vi "CRYProbe Window Change.vi"(6 "Update Index":i32[](array[numeric]), 8 "Type":enum16{"Curves", "Values", "Results", "WFM"}(ring), 9 "Close Names":string[](array[string]), 10 "Update Names":string[](array[string]), 11 "Probe Type":string) -> ()   [LabVIEW 2013]
uses:
  Global/CRYCurve Library Global.vi
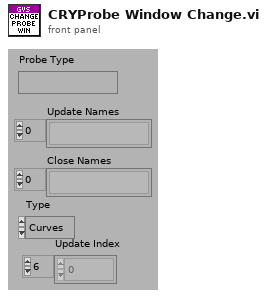
[diagram p1: front panel]
types:
  T1 = cluster{"Type Name":string, "Data Name":string, "Probe VIRef Number":i32, "Probe VIRef":refnum<vi>}[]
  T2 = cluster{"Type Name":string, "Data Name":string, "Probe VIRef Number":i32, "Probe VIRef":refnum<vi>}
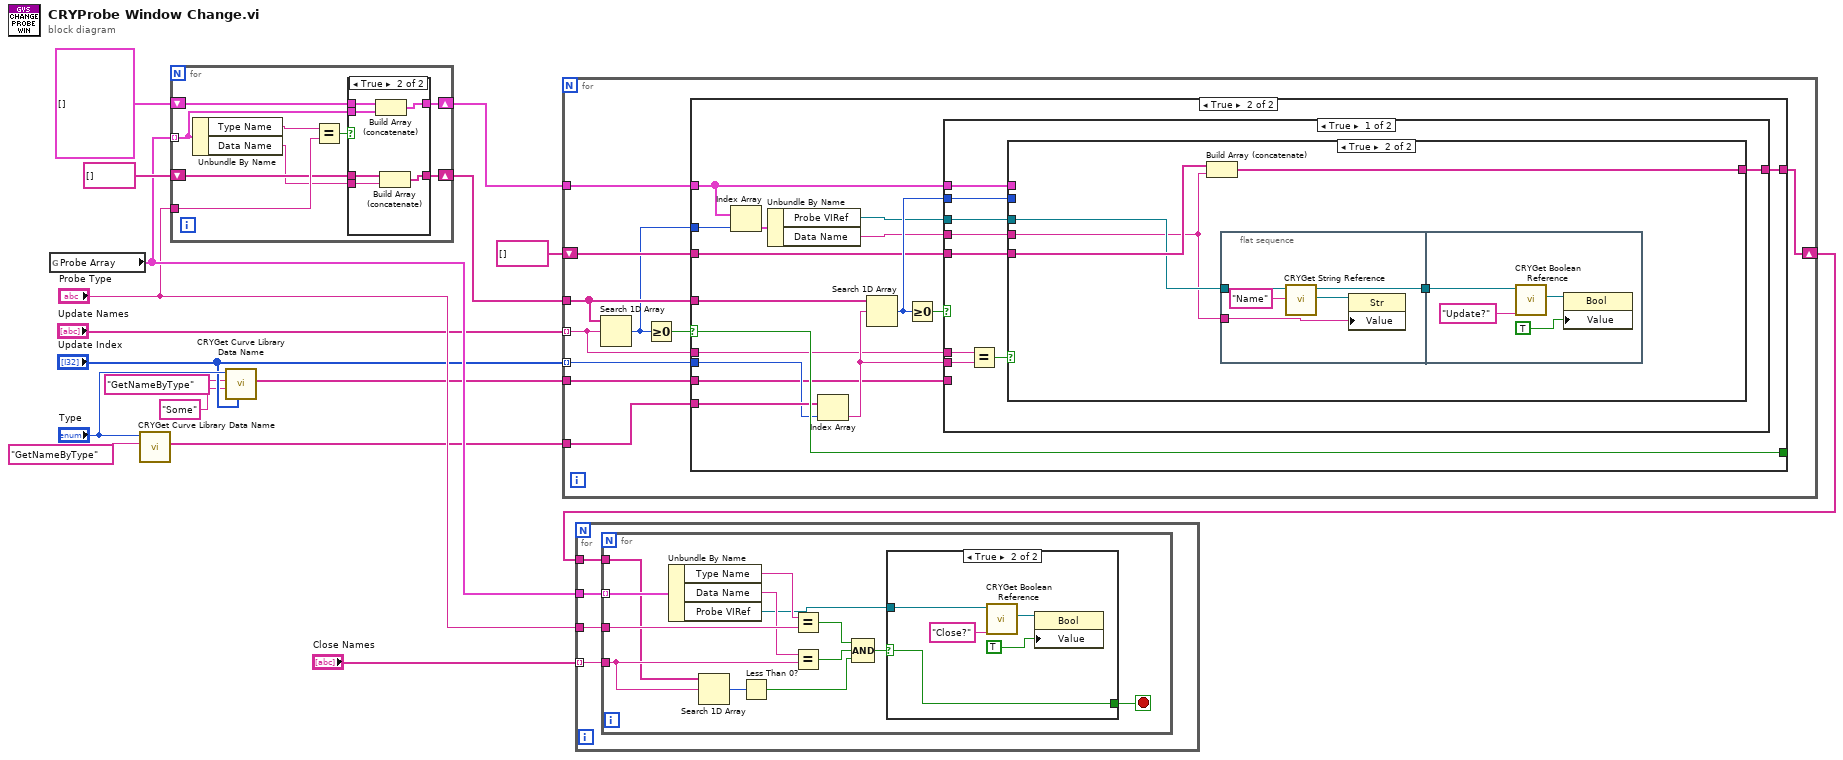
[diagram p0: block diagram]
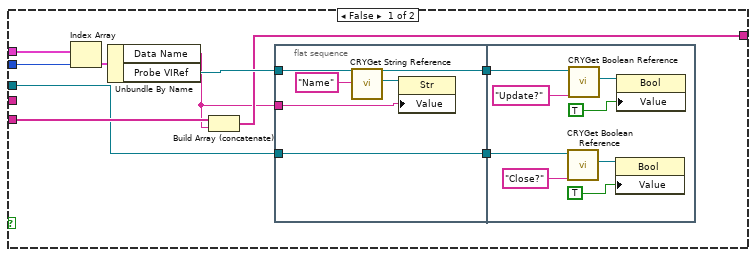
[diagram p5: hidden frame]
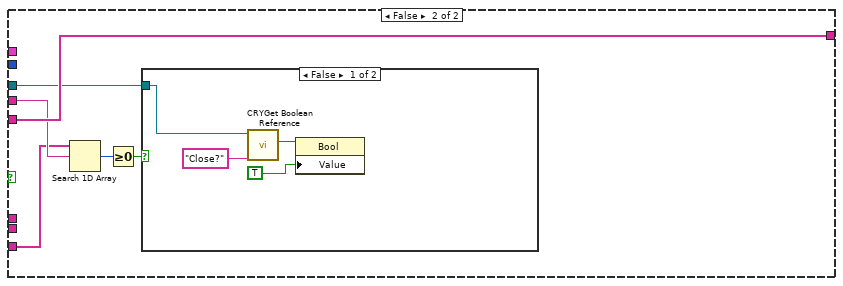
[diagram p6: hidden frame]
diagram:
  n1 = global read "CRYCurve Library Global.vi" "Probe Array"() -> (w14:T1)
  n2 = call "CRYGet Curve Library Data Name.vi"("sAction"="GetNameByType", "Type"="Type") -> ("sNames"=w8:string[])  [unwired: 4 in, 5 out]
  n3 = for {
    tunnel: w14 -> [w22] mode=indexing
    tunnel: "Probe Type" -> [w25]
    shift-right: [w21] -> w13
    shift-left: T1 [] ("Probe Array") -> [w23]
    shift-right: [w18] -> w12
    shift-left: string[] [] -> [w20]
    n4 = Unbundle By Name(w22) -> ("Type Name"=w26:string, "Data Name"=w19:string)
    n5 = Equal?(x=w26, y=w25) -> (x = y?=w24:bool)
    n6 = case shown="True" w24 {
      tunnel: w23 -> [w28 w34]
      tunnel: w22 -> [_ w33]
      tunnel: [w28 w32] -> w21
      tunnel: w20 -> [w27 w31]
      tunnel: w19 -> [_ w30]
      tunnel: [w27 w29] -> w18
      frame False {
      }
      frame True {
        n7 = Build Array (concatenate)(w34, w33) -> (w32:T1)
        n8 = Build Array (concatenate)(w31, w30) -> (w29:string[])
      }
    }
  }
  n9 = call "CRYGet Curve Library Data Name.vi"("nData"="Update Index", "sOption"="Some" ("sAction"), "sAction"="GetNameByType", "Type"="Type") -> ("sNames"=w5:string[])  [unwired: 2 in, 5 out]
  n10 = for {
    tunnel: "Update Names" -> [w38] mode=indexing
    tunnel: w13 -> [w37]
    tunnel: w12 -> [w40]
    shift-right: [w43] -> w9
    shift-left: string[] [] -> [w44]
    tunnel: "Update Index" -> [w42] mode=indexing
    tunnel: w8 -> [w41]
    tunnel: w5 -> [w35]
    n11 = Search 1D Array(1D array=w40, element=w38) -> (index of element=w36:i32)  [unwired: 1 in]
    n12 = Greater Or Equal To 0?(x=w36) -> (x >= 0?=w39:bool)
    n13 = case shown="True" w39 {
      selector: w39 -> [w46 w60]
      tunnel: [w46 w60] -> _
      tunnel: w40 -> [_ w62]
      tunnel: w37 -> [_ w50]
      tunnel: w44 -> [w45 w59]
      tunnel: [w45 w58] -> w43
      tunnel: w41 -> [_ w56]
      tunnel: w42 -> [_ w55]
      tunnel: w38 -> [_ w53]
      tunnel: w36 -> [_ w51]
      tunnel: w35 -> [_ w47]
      frame False {
      }
      frame True {
        n14 = Index Array(array=w50, index=w51) -> (element=w52:T2)
        n15 = Unbundle By Name(w52) -> ("Probe VIRef"=w49:refnum<vi>, "Data Name"=w48:string)
        n16 = Index Array(array=w56, index=w55) -> (element=w54:string)
        n17 = Search 1D Array(1D array=w62, element=w54) -> (index of element=w61:i32)  [unwired: 1 in]
        n18 = Greater Or Equal To 0?(x=w61) -> (x >= 0?=w57:bool)
        n19 = case shown="True" w57 {
          tunnel: w50 -> [w70 _]
          tunnel: w61 -> [w65 _]
          tunnel: w59 -> [w69 w115]
          tunnel: [w68 w115] -> w58
          tunnel: w54 -> [w67 _]
          tunnel: w53 -> [w66 _]
          tunnel: w49 -> [w64 w111]
          tunnel: w48 -> [w63 w114]
          tunnel: w47 -> [_ w110]
          frame True {
            n20 = Equal?(x=w66, y=w67) -> (x = y?=w71:bool)
            n21 = case shown="True" w71 {
              tunnel: w70 -> [w77 _]
              tunnel: w69 -> [w76 w99]
              tunnel: [w75 w98] -> w68
              tunnel: w65 -> [w74 _]
              tunnel: w64 -> [w73 w97]
              tunnel: w63 -> [_ w96]
              frame False {
                n22 = Index Array(array=w77, index=w74) -> (element=w79:T2)
                n23 = Unbundle By Name(w79) -> ("Data Name"=w72:string, "Probe VIRef"=w78:refnum<vi>)
                n24 = Build Array (concatenate)(w76, w72) -> (w75:string[])
                n25 = flat-sequence {
                  tunnel: w78 -> [w84]
                  tunnel: [w83] -> w81
                  tunnel: [w87] -> w80
                  tunnel: w73 -> [w87]
                  tunnel: w72 -> [w82]
                  tunnel: w81 -> [w92]
                  tunnel: w80 -> [w89]
                  frame #0 {
                    n26 = call "CRYGet String Reference.vi"("Label Name"="Name", "VI Refnum"=w84) -> ("String Ref Out"=w85:refnum<vi>, "VI Refnum Out"=w83:refnum<vi>)  [unwired: 8 out]
                    n27 = property class="Str"(reference=w85, "Value"=w82) -> ()  [unwired: 1 in, 2 out]
                  }
                  frame #1 {
                    n28 = call "CRYGet Boolean Reference.vi"("Label Name"="Close?", "VI Refnum"=w89) -> ("Boolean Ref"=w88:refnum<vi>)  [unwired: 9 out]
                    n29 = call "CRYGet Boolean Reference.vi"("Label Name"="Update?", "VI Refnum"=w92) -> ("Boolean Ref"=w94:refnum<vi>)  [unwired: 9 out]
                    n30 = property class="Bool"(reference=w88, "Value"=TRUE) -> ()  [unwired: 1 in, 2 out]
                    n31 = property class="Bool"(reference=w94, "Value"=TRUE) -> ()  [unwired: 1 in, 2 out]
                  }
                }
              }
              frame True {
                n32 = Build Array (concatenate)(w99, w96) -> (w98:string[])
                n33 = flat-sequence {
                  tunnel: w97 -> [w103]
                  tunnel: [w102] -> w100
                  tunnel: w96 -> [w101]
                  tunnel: w100 -> [w106]
                  frame #0 {
                    n34 = call "CRYGet String Reference.vi"("Label Name"="Name", "VI Refnum"=w103) -> ("String Ref Out"=w104:refnum<vi>, "VI Refnum Out"=w102:refnum<vi>)  [unwired: 8 out]
                    n35 = property class="Str"(reference=w104, "Value"=w101) -> ()  [unwired: 1 in, 2 out]
                  }
                  frame #1 {
                    n36 = call "CRYGet Boolean Reference.vi"("Label Name"="Update?", "VI Refnum"=w106) -> ("Boolean Ref"=w108:refnum<vi>)  [unwired: 9 out]
                    n37 = property class="Bool"(reference=w108, "Value"=TRUE) -> ()  [unwired: 1 in, 2 out]
                  }
                }
              }
            }
          }
          frame False {
            n38 = Search 1D Array(1D array=w110, element=w114) -> (index of element=w113:i32)  [unwired: 1 in]
            n39 = Greater Or Equal To 0?(x=w113) -> (x >= 0?=w112:bool)
            n40 = case shown="False" w112 {
              tunnel: w111 -> [w116 _]
              frame False {
                n41 = call "CRYGet Boolean Reference.vi"("Label Name"="Close?", "VI Refnum"=w116) -> ("Boolean Ref"=w117:refnum<vi>)  [unwired: 9 out]
                n42 = property class="Bool"(reference=w117, "Value"=TRUE) -> ()  [unwired: 1 in, 2 out]
              }
              frame True {
              }
            }
          }
        }
      }
    }
  }
  n43 = for {
    tunnel: w14 -> [w123]
    tunnel: "Probe Type" -> [w122]
    tunnel: "Close Names" -> [w121] mode=indexing
    tunnel: w9 -> [w120]
    n44 = for {
      tunnel: w123 -> [w136] mode=indexing
      tunnel: w122 -> [w134]
      tunnel: w121 -> [w127]
      tunnel: w120 -> [w124]
      stop <- w128 stop-if-true
      n45 = Unbundle By Name(w136) -> ("Type Name"=w135:string, "Data Name"=w133:string, "Probe VIRef"=w130:refnum<vi>)
      n46 = Search 1D Array(1D array=w124, element=w127) -> (index of element=w126:i32)  [unwired: 1 out]
      n47 = Less Than 0?(x=w126) -> (x < 0?=w125:bool)
      n48 = Equal?(x=w135, y=w134) -> (x = y?=w131:bool)
      n49 = Equal?(x=w133, y=w127) -> (x = y?=w132:bool)
      n50 = Compound Arithmetic op=AND(w131, w132, w125) -> (w129:bool)
      n51 = case shown="True" w129 {
        selector: w129 -> [w137 w142]
        tunnel: w130 -> [_ w138]
        tunnel: [w137 w142] -> w128
        frame False {
        }
        frame True {
          n52 = call "CRYGet Boolean Reference.vi"("Label Name"="Close?", "VI Refnum"=w138) -> ("Boolean Ref"=w140:refnum<vi>)  [unwired: 9 out]
          n53 = property class="Bool"(reference=w140, "Value"=TRUE) -> ()  [unwired: 1 in, 2 out]
        }
      }
    }
  }
